vi "Robot_glass_control__computer.vi"() -> ()   [LabVIEW 2012]
uses:
  <vilib>/NXT/Block Support/NXT_MessageMailbox.ctl
  <vilib>/httpClient/LabVIEWHTTPClient.lvlib
panel:
  out "ajax response":string
  in  "request":string="http://narek.galstyan1996.student.tumo.org/LabView/?LabView"
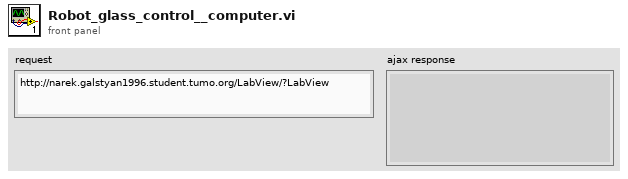
[diagram p1: front panel]
types:
  T1 = typedef "NXT_MessageMailbox.ctl" = u8
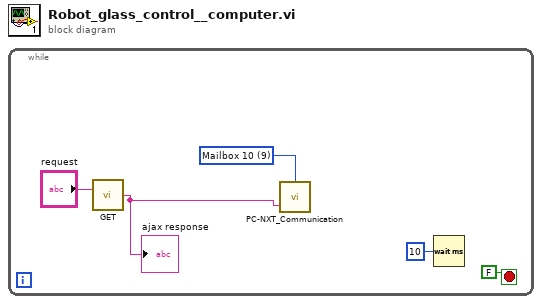
[diagram p0: block diagram]
diagram:
  n1 = while {
    stop <- FALSE stop-if-true
    w2 = T1 9 items=["Mailbox 1", "Mailbox 2", "Mailbox 3", "Mailbox 4", "Mailbox 5", "Mailbox 6", "Mailbox 7", "Mailbox 8", "Mailbox 9", "Mailbox 10"] ("Mailbox (Mailbox 1)")
    n2 = call <vilib>:"GET.vi"("url"="request") -> ("body"=w3:string)  [unwired: 11 in, 3 out]
    "ajax response" <- w3
    n3 = call <vilib>:"PC-NXT_Communication.vi"("Message"=w3, "Mailbox (Mailbox 1)"=w2) -> ()  [unwired: 2 in, 1 out]
    n4 = Wait (ms)(milliseconds to wait=u32 10) -> ()  [unwired: 1 out]
  }
